vi "Teleop.vi"(10 "Match Info":T1={"Autonomous Elapsed Seconds"=0.0, "TeleOp Elapsed Seconds"=0.0, "Disabled Elapsed Seconds"=0.0, "Visited Autonomous"=FALSE, "Visited TeleOp"=FALSE, "Visited Disabled"=FALSE, "Autonomous Settings"={"Autonomous Style"=enum."Independent", "VI Refnum"=refnum}}, 11 "Call Context":T2) -> ()   [LabVIEW 2016]
doc: "This VI is called for each TeleOp packet received from the DS where the robot is not disabled. It is often used to read from the joysticks and update I/O or to update setpoints for timed control loops. It should complete and return within 20 milliseconds or it may miss DS packets."
uses:
  <vilib>/Rock Robotics/WPI/DriverStation/WPI_DriverStationDerivedRobotMode.ctl
  <vilib>/Rock Robotics/WPI/DriverStation/WPI_DriverStationMatch Info.ctl
  <vilib>/Rock Robotics/Network Tables/NT Read Boolean.vi
  <vilib>/Rock Robotics/Network Tables/NT Read Number.vi
  Globals/Constantes.vi
  Globals/InputValues.vi
  Globals/Globals.vi
panel:
  in  "Dont block":bool
  out "Sample Slider 0":dbl(slide) scale=0.0..5.0
  out "Sample Boolean 1":bool
  out "Sample Boolean 0":bool
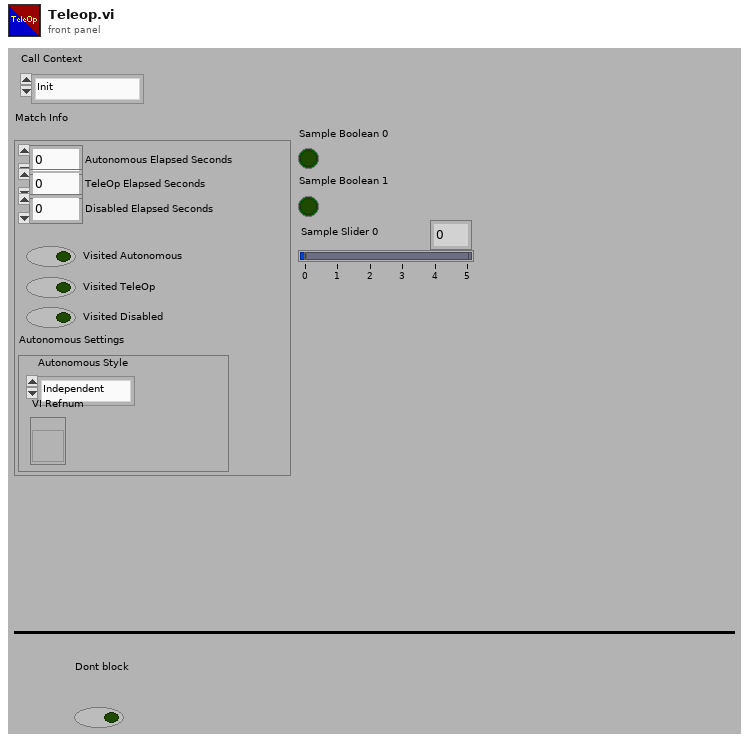
[diagram p1: front panel]
types:
  T1 = typedef "WPI_DriverStationMatch Info.ctl" = cluster{"Autonomous Elapsed Seconds":dbl, "TeleOp Elapsed Seconds":dbl, "Disabled Elapsed Seconds":dbl, "Visited Autonomous":bool, "Visited TeleOp":bool, "Visited Disabled":bool, "Autonomous Settings":cluster{"Autonomous Style":enum16{"Iterative", "Independent"}, "VI Refnum":refnum<vi>}}
  T2 = typedef "WPI_DriverStationDerivedRobotMode.ctl" = enum16{"Init", "Execute", "Stop"}
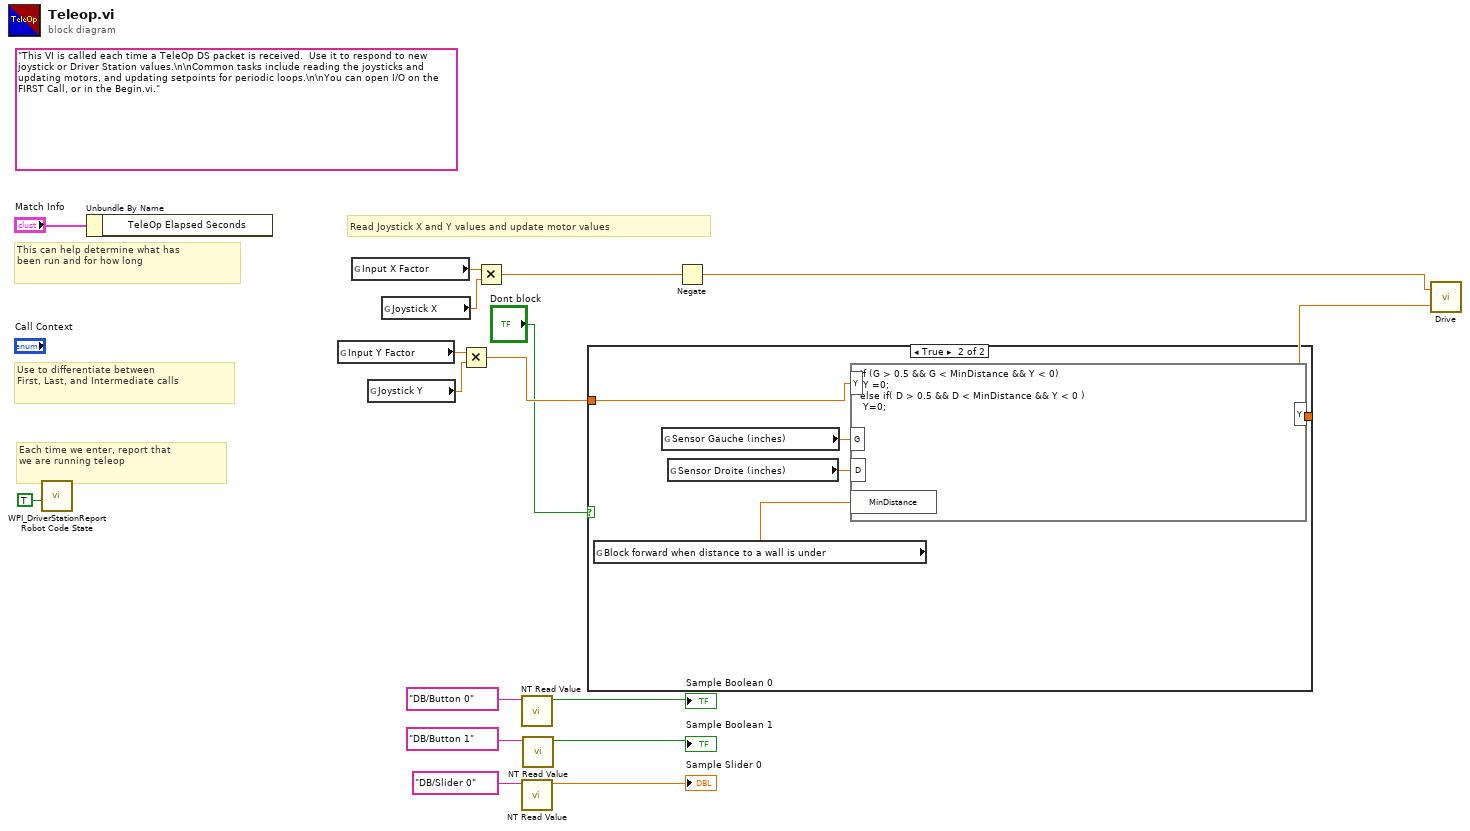
[diagram p0: block diagram]
diagram:
  (unwired) "This VI is called each time a TeleOp DS packet is received.  Use it to respond to new joystick or Driver Station values.\n\nCommon tasks include reading the joysticks and updating motors, and updating setpoints for periodic loops.\n\nYou can open I/O on the FIRST Call, or in the Begin.vi."
  # "Each time we enter, report that\nwe are running teleop"
  # "Use to differentiate between\nFirst, Last, and Intermediate calls"
  # "This can help determine what has\nbeen run and for how long"
  # "Read Joystick X and Y values and update motor values"
  n1 = call <vilib>:"WPI_DriverStationReport Robot Code State.vi"("TeleOp"=TRUE ("Autonomous")) -> ()  [unwired: 10 in, 1 out]
  n2 = Unbundle By Name("Match Info") -> ()  [unwired: 1 out]
  n3 = global read "Constantes.vi" "Input Y Factor"() -> (w7:dbl)
  n4 = global read "Constantes.vi" "Input X Factor"() -> (w8:dbl)
  n5 = global read "InputValues.vi" "Joystick Y"() -> (w6:dbl)
  n6 = global read "InputValues.vi" "Joystick X"() -> (w5:dbl)
  n7 = Multiply(x=w7, y=w6) -> (x*y=w9:dbl)
  n8 = Multiply(x=w8, y=w5) -> (x*y=w4:dbl)
  n9 = call-poly <vilib>:"NT Read Value.vi"("Name"="DB/Button 0" ("refnum name")) -> ("Boolean"=→"Sample Boolean 0":bool)  [unwired: 9 in, 1 out]
  n10 = call-poly <vilib>:"NT Read Value.vi"("Name"="DB/Slider 0" ("refnum name")) -> ("Numeric"=→"Sample Slider 0":dbl)  [unwired: 9 in, 1 out]
  n11 = call-poly <vilib>:"NT Read Value.vi"("Name"="DB/Button 1" ("refnum name")) -> ("Boolean"=→"Sample Boolean 1":bool)  [unwired: 9 in, 1 out]
  n12 = case shown="True" "Dont block" {
    tunnel: w9 -> [w18 w23]
    tunnel: [w18 w19] -> w2
    frame False {
    }
    frame True {
      n13 = global read "Constantes.vi" "Block forward when distance to a wall is under"() -> (w20:dbl)
      n14 = global read "Globals.vi" "Sensor Gauche (inches)"() -> (w22:dbl)
      n15 = global read "Globals.vi" "Sensor Droite (inches)"() -> (w21:dbl)
      n16 = formula code="if (G > 0.5 && G < MinDistance && Y < 0)\n Y =0;\nelse if( D > 0.5 && D < MinDistance && Y < 0 )\n Y=0;"("G"=w22, "D"=w21, "Y"=w23, "MinDistance"=w20) -> ("Y"=w19:dbl)
    }
  }
  n17 = Negate(x=w4) -> (-x=w1:dbl)
  n18 = call "Drive.vi"("Y (Forward)"=w2, "X (Rotation)"=w1) -> ()  [unwired: 1 in]
